vi "Obtain Actual Voltage.vi"(8 "Error In":errorcluster, 10 "Error Percentage":dbl, 11 "Mode in":refnum<class "Mode.lvclass">) -> (0 "Error Out":errorcluster, 3 "Mode out":refnum<class "Mode.lvclass">)   [LabVIEW 2023, in "Mode.lvclass"]
uses:
  Mode.lvclass
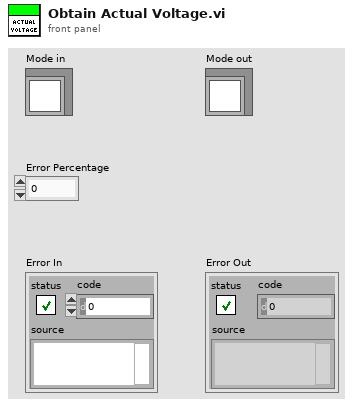
[diagram p1: front panel]
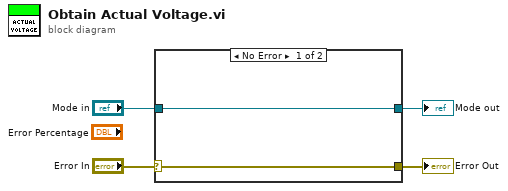
[diagram p0: block diagram]
diagram:
  n1 = case shown="No Error" "Error In" {
    selector: "Error In" -> [w5 w8]
    tunnel: [w5 w8] -> w3
    tunnel: [w6 w7] -> w1
    tunnel: "Mode in" -> [w6 w7]
    frame No Error {
    }
    frame Error {
    }
  }
  "Error Out" <- w3
  "Mode out" <- w1
